vi "plot_loadYoung.vi"(0 "Output Path":path=path "C:/WXT-ORG/Data", 3 "Young Prefix":string="Young", 9 "Time":timestamp, 11 "Offset (hrs)":dbl) -> (8 "Loaded Data Array":dbl[][](array[numeric]), 10 "Last Tips Value":dbl, 15 "Timestamp":dbl[](array[numeric]))   [LabVIEW 2018]
uses:
  <vilib>/Utility/file.llb/Read From Spreadsheet File (DBL).vi
panel:
  out "YNG Wind Gusts":dbl[](array[numeric])
  out "YNG Rain Fall":dbl[](array[numeric])
  out "YNG Rain Rate":dbl[](array[numeric])
  out "YNG Tips":dbl[](array[numeric])
  out "YNG Timestamp":dbl[](array[numeric])
  out "YNG Wind Speed":dbl[](array[numeric])
  out "YNG Wind Direction":dbl[](array[numeric])
  out "YNG Temperature":dbl[](array[numeric])
  out "YNG Humidity 2":dbl[](array[numeric])
  out "YNG Pressure":dbl[](array[numeric])
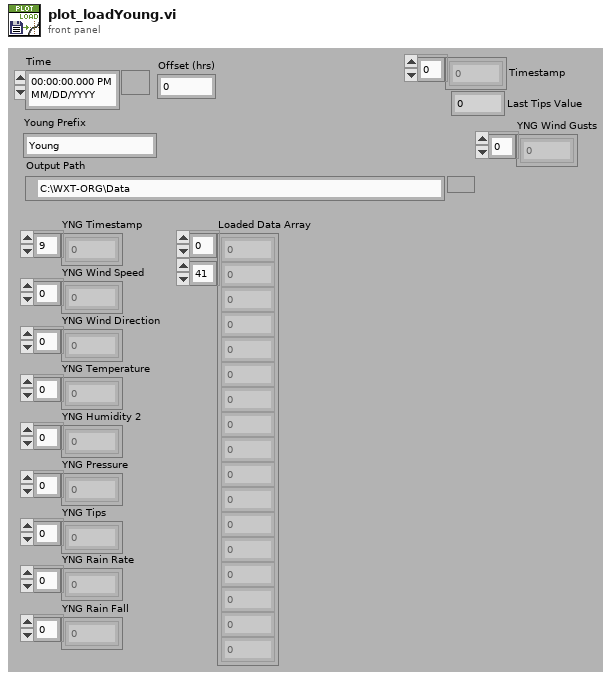
[diagram p1: front panel]
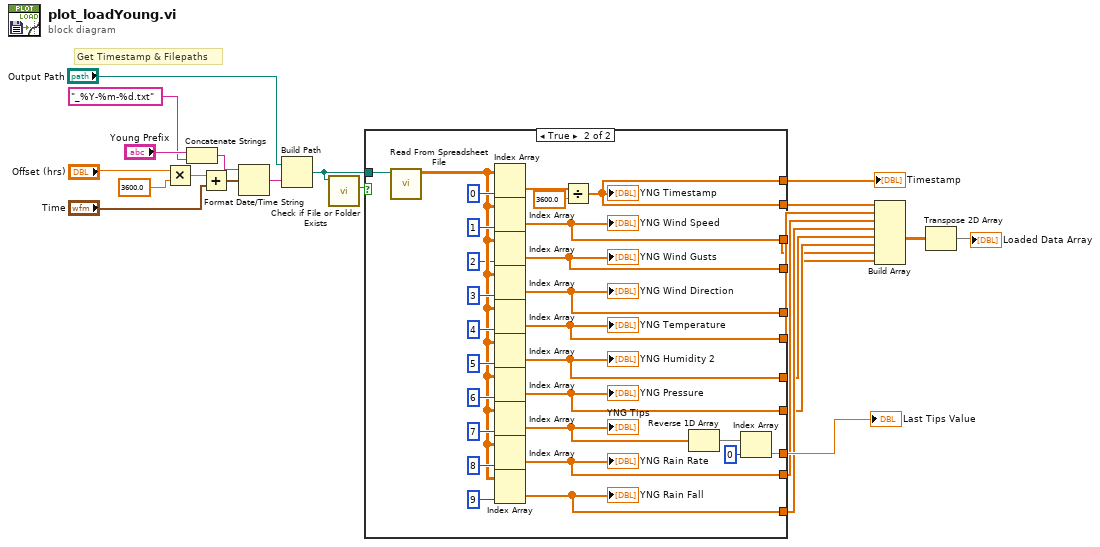
[diagram p0: block diagram]
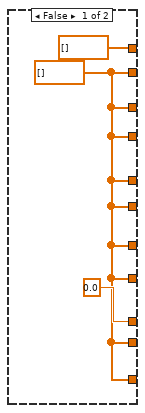
[diagram p2: hidden frame]
diagram:
  # "Get Timestamp & Filepaths"
  n1 = Multiply(x="Offset (hrs)", y=3600.0) -> (x*y=w23:dbl)
  n2 = Concatenate Strings("Young Prefix", "_%Y-%m-%d.txt" ("string")) -> (w18:string)
  n3 = Add(x=w23, y="Time") -> (x+y=w17:timestamp)
  n4 = Format Date/Time String(time format string (%c)=w18, seconds (now)=w17) -> (date/time string=w16:string)  [unwired: 1 in]
  n5 = Build Path(base path="Output Path", name or relative path=w16) -> (appended path=w11:path)
  n6 = call <vilib>:"Check if File or Folder Exists.vi"("path"=w11) -> ("file or folder exists?"=w14:bool)  [unwired: 8 in, 2 out]
  n7 = case shown="True" w14 {
    tunnel: w11 -> [_ w48]
    tunnel: [w25 w32] -> w9
    tunnel: [w25 w47] -> w3
    tunnel: [w25 w46] -> _
    tunnel: [w25 w40] -> w8
    tunnel: [w25 w39] -> w6
    tunnel: [w25 w38] -> w5
    tunnel: [w25 w37] -> w4
    tunnel: [w25 w36] -> w7
    tunnel: [0.0 w33] -> w10
    tunnel: [dbl[] [] w32] -> w2
    tunnel: [w25 w29] -> w1
    frame False {
      w25 = dbl[] [] ("all rows")
    }
    frame True {
      n8 = call-poly <vilib>:"Read From Spreadsheet File.vi"("file path (dialog if empty)"=w48) -> ("all rows"=w30:dbl[][])  [unwired: 6 in, 4 out]
      n9 = Index Array(array=w30, index (col)=0 ("disabled index (col)")) -> (element=w44:dbl[])  [unwired: 1 in]
      n10 = Index Array(array=w30, index (col)=1 ("disabled index (col)")) -> (element=w47:dbl[])  [unwired: 1 in]
      "YNG Wind Speed" <- w47
      n11 = Index Array(array=w30, index (col)=2 ("disabled index (col)")) -> (element=w29:dbl[])  [unwired: 1 in]
      "YNG Wind Gusts" <- w29
      n12 = Index Array(array=w30, index (col)=3 ("disabled index (col)")) -> (element=w46:dbl[])  [unwired: 1 in]
      "YNG Wind Direction" <- w46
      n13 = Index Array(array=w30, index (col)=4 ("disabled index (col)")) -> (element=w40:dbl[])  [unwired: 1 in]
      "YNG Temperature" <- w40
      n14 = Index Array(array=w30, index (col)=5 ("disabled index (col)")) -> (element=w38:dbl[])  [unwired: 1 in]
      "YNG Humidity 2" <- w38
      n15 = Index Array(array=w30, index (col)=6 ("disabled index (col)")) -> (element=w37:dbl[])  [unwired: 1 in]
      "YNG Pressure" <- w37
      n16 = Index Array(array=w30, index (col)=7 ("disabled index (col)")) -> (element=w35:dbl[])  [unwired: 1 in]
      "YNG Tips" <- w35
      n17 = Index Array(array=w30, index (col)=8 ("disabled index (col)")) -> (element=w36:dbl[])  [unwired: 1 in]
      "YNG Rain Rate" <- w36
      n18 = Index Array(array=w30, index (col)=9 ("disabled index (col)")) -> (element=w39:dbl[])  [unwired: 1 in]
      "YNG Rain Fall" <- w39
      n19 = Divide(x=w44, y=3600.0) -> (x/y=w32:dbl[])
      "YNG Timestamp" <- w32
      n20 = Reverse 1D Array(array=w35) -> (reversed array=w34:dbl[])
      n21 = Index Array(array=w34, index=0) -> (element=w33:dbl)
    }
  }
  "Timestamp" <- w2
  "Last Tips Value" <- w10
  n22 = Build Array(w9, w8, w7, w6, w5, w4, w3, w1) -> (w12:dbl[][])
  n23 = Transpose 2D Array(2D array=w12) -> (transposed array=→"Loaded Data Array":dbl[][])
